vi "Input_IR.vi"(11 "Analog Input":dbl) -> (3 "Distance (in)":dbl)   [LabVIEW 2012]
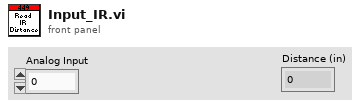
[diagram p1: front panel]
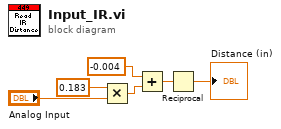
[diagram p0: block diagram]
diagram:
  n1 = Multiply(x=0.183, y="Analog Input") -> (x*y=w3:dbl)
  n2 = Add(x=-0.004, y=w3) -> (x+y=w4:dbl)
  n3 = Reciprocal(x=w4) -> (1/x=→"Distance (in)":dbl)
